vi "DMM data.vi"(0 "VISA resource name":refnum<visa-resource-name>, 1 "error in (no error)":errorcluster {"code" format="%.0x"}) -> (2 "VISA resource name out":refnum<visa-resource-name>, 3 "Voltage":dbl, 4 "error out":errorcluster {"code" format="%.0x"})   [LabVIEW 2015]
uses:
  <instrlib>/Hameg DMM/Hameg DMM.lvlib
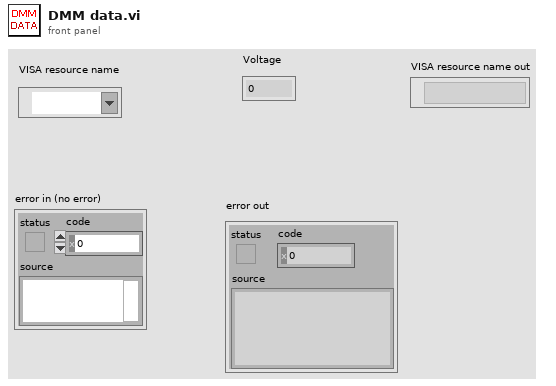
[diagram p1: front panel]
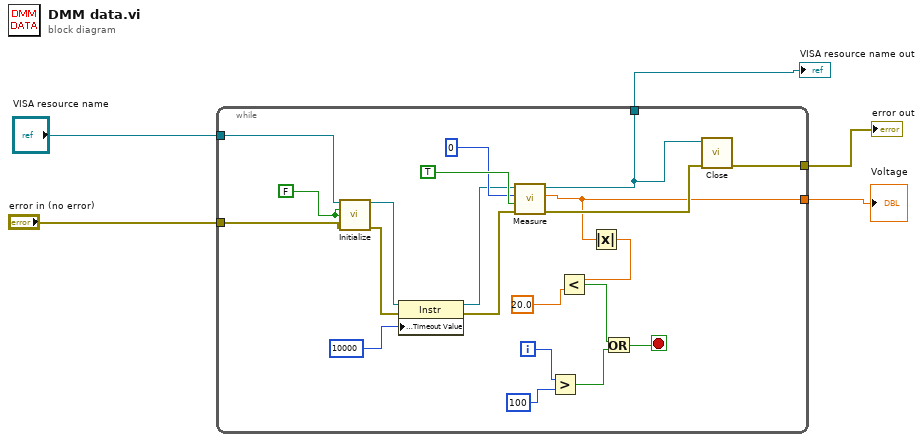
[diagram p0: block diagram]
diagram:
  n1 = while {
    tunnel: [w14] -> w5
    tunnel: "VISA resource name" -> [w22]
    tunnel: "error in (no error)" -> [w21]
    tunnel: [w6] -> w2
    tunnel: [w7] -> w1
    i -> [w16]
    stop <- w17 stop-if-true
    w23 = FALSE
    n2 = call <instrlib>:"Initialize.vi"("VISA resource name"=w22, "ID Query (T: Check)"=w23, "Reset (T: Reset)"=w23, "error in (no error)"=w21) -> ("VISA resource name out"=w11:refnum<visa-resource-name>, "error out"=w10:errorcluster)  [unwired: 10 in]
    n3 = property class="Instr"(reference=w11, error in=w10, "General Settings:Timeout Value"=u32 10000) -> (reference out=w9:refnum<visa-resource-name>, error out=w8:errorcluster)
    n4 = call <instrlib>:"Measure.vi"("error in (no error)"=w8, "Autorange (T: On)"=TRUE, "Function (0: DC Voltage)"=0, "VISA resource name"=w9) -> ("error out"=w15:errorcluster, "Measurement Value"=w14:dbl, "VISA resource name out"=w7:refnum<visa-resource-name>)  [unwired: 5 in]
    n5 = Greater?(x=w16, y=100) -> (0:w18:bool)
    n6 = Absolute Value(x=w14) -> (abs(x)=w13:dbl)
    n7 = Less?(x=w13, y=20.0) -> (x < y?=w19:bool)
    n8 = Or(x=w19, y=w18) -> (x .or. y?=w17:bool)
    n9 = call <instrlib>:"Close.vi"("error in (no error)"=w15, "VISA resource name"=w7) -> ("error out"=w6:errorcluster)  [unwired: 9 in]
  }
  "error out" <- w2
  "Voltage" <- w5
  "VISA resource name out" <- w1
